vi "SMO.Dictionary.Variant.TestLauncher.vi"() -> ()   [LabVIEW 2013, in "SMO.Dictionary.lvlib" / "SMO.Dictionary.Variant.lvclass"]
uses:
  SMO.Dictionary.Variant.lvclass
  <vilib>/JKI/JKI SMO/SMO/Typedefs/SMOState --Enum.ctl
  <vilib>/JKI/JKI SMO/SMO/SMO.lvclass/SMO.ctl
  <vilib>/JKI/JKI SMO/SMO/Private/ReftoDVR--SMO.vi
  <vilib>/JKI/JKI SMO/SMO/SMO.lvclass
  SMO.Dictionary/SMO.Dictionary.lvclass
panel:
  out "deleted":bool
  in  "Delete String":bool
  out "echo":string
  out "Values":variant[](array[variant])
  in  "string":string
  in  "Update String":bool
  out "SMO State":T1
  out "error out":errorcluster
  in  "Stop":bool
  # "Variant Attributes Dictionary Test Launcher"
  # "For instructions on how to use the JKI State Machine Objects, examples and video tutorials, visit:\nhttp://jki.net/state-machine-objects/\n\nJKI State Machine Objects™\nhttp://jki.net/state-machine-objects/\nCopyright (C) 2005-2015, JKI <info@jki.net>\nALL RIGHTS RESERVED"
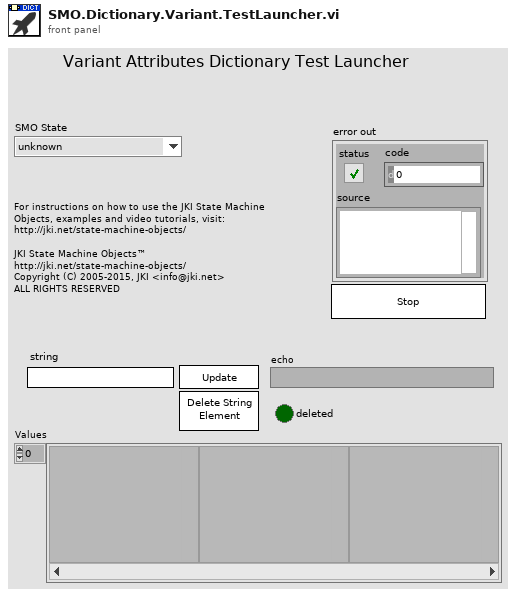
[diagram p1: front panel]
types:
  T1 = typedef "SMO.lvclass/SMOState --Enum.ctl" = enum16{"unknown", "Created", "Started", "Stopped"}
  T2 = typedef "SMO.lvclass/Public Events.ctl" = cluster{"Error":refnum<user-event>, "State":refnum<user-event>, "Reserve State":refnum<user-event>}
  T3 = typedef "SMO.Dictionary.lvlib/SMO.Dictionary.lvclass/PublicEvents--Cluster.ctl" = cluster{"Cleared":refnum<user-event>, "Deleted":refnum<user-event>, "Updated":refnum<user-event>}
  T4 = cluster{"Event Registration Refnum":refnum<event-registration>}
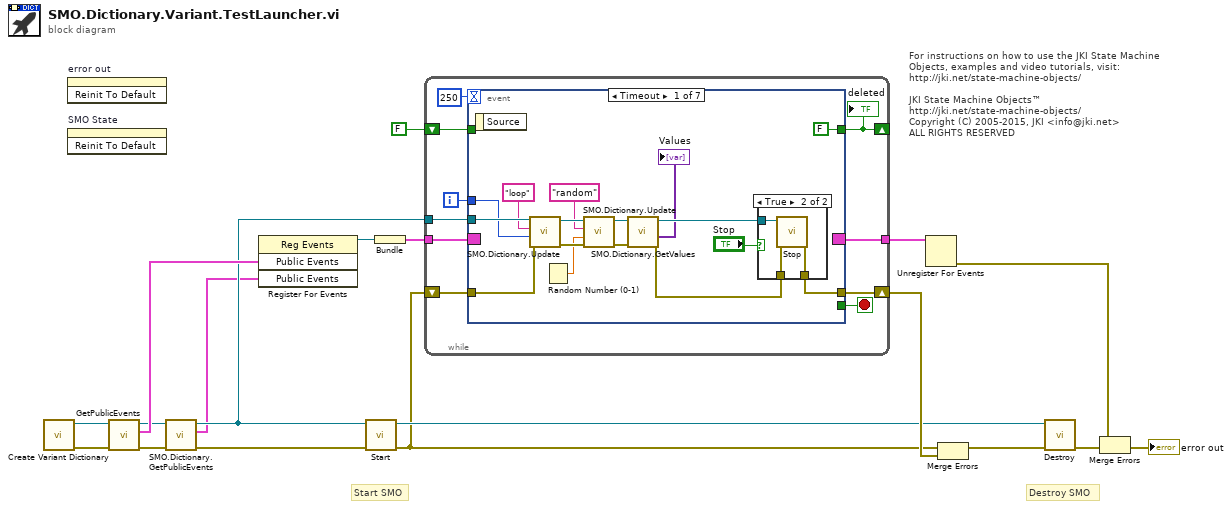
[diagram p0: block diagram]
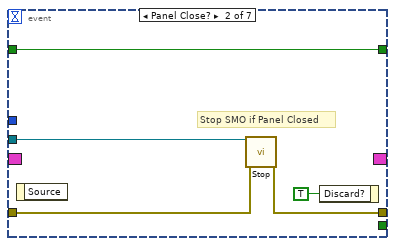
[diagram p3: hidden frame]
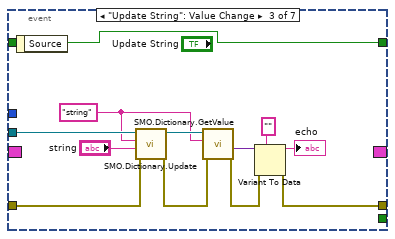
[diagram p4: hidden frame]
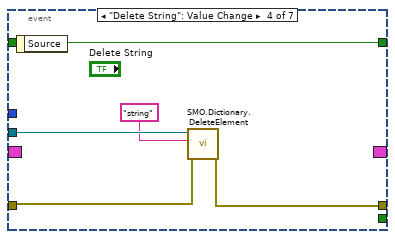
[diagram p5: hidden frame]
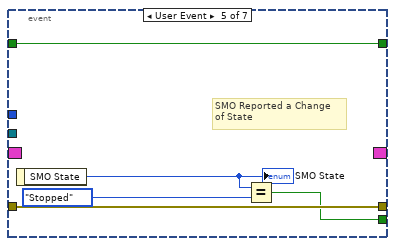
[diagram p6: hidden frame]
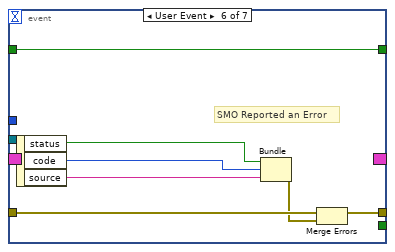
[diagram p7: hidden frame]
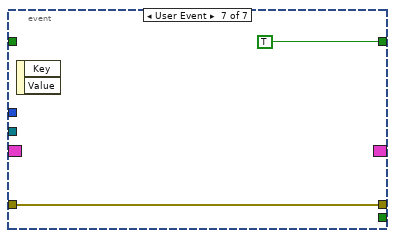
[diagram p8: hidden frame]
diagram:
  # "For instructions on how to use the JKI State Machine Objects, examples and video tutorials, visit:\nhttp://jki.net/state-machine-objects/\n\nJKI State Machine Objects™\nhttp://jki.net/state-machine-objects/\nCopyright (C) 2005-2015, JKI <info@jki.net>\nALL RIGHTS RESERVED"
  # "Start SMO"
  # "Destroy SMO"
  n1 = call "Create Variant Dictionary.vi"() -> ("error out"=w2:errorcluster, "SMO.Dictionary.Variant out"=w3:refnum<class "SMO.Dictionary.Variant.lvclass">)  [unwired: 9 in, 1 out]
  n2 = invoke on="error out" class="Clust (strict)" method="Reinit To Default"() -> ()  [unwired: 3 in, 3 out]
  n3 = invoke on="SMO State" class="Enum (strict)" method="Reinit To Default"() -> ()  [unwired: 3 in, 3 out]
  n4 = call <vilib>:"GetPublicEvents.vi"("error in (no error)"=w2, "SMO"=w3) -> ("error out"=w8:errorcluster, "Public Events"=w12:T2, "SMO out"=w10:refnum<class "SMO.Dictionary.Variant.lvclass">)  [unwired: 7 in]
  n5 = call "SMO.Dictionary.GetPublicEvents.vi"("error in (no error)"=w8, "SMO.Dictionary in"=w10) -> ("error out"=w7:errorcluster, "Public Events"=w6:T3, "SMO.Dictionary out"=w9:refnum<class "SMO.Dictionary.Variant.lvclass">)  [unwired: 7 in]
  n6 = register-events(w12, w6) -> (reference out=w11:refnum<event-registration>)  [unwired: 2 in, 1 out]
  n7 = call <vilib>:"Start.vi"("error in (no error)"=w7, "SMO"=w9) -> ("error out"=w4:errorcluster, "SMO out"=w5:refnum<class "SMO.Dictionary.Variant.lvclass">)  [unwired: 8 in]
  n8 = Bundle("Event Registration Refnum"=w11) -> (w18:T4)  [unwired: 1 in]
  n9 = while {
    shift-right: [w28] -> w17
    shift-left: w4 -> [w27]
    tunnel: w18 -> [w26]
    tunnel: [w25] -> w19
    tunnel: w9 -> [w24]
    shift-right: [w20] -> _
    shift-left: FALSE -> [w21]
    i -> [w22]
    stop <- w29 stop-if-true
    n10 = event shown="[0] Timeout" {
      selector: w26 -> [_ _ _ _ _ _ _]
      dyn-events: [_ _ _ _ _ _ _] -> w25
      timeout: 250 -> [_ _ _ _ _ _ _]
      tunnel: [_ _ _ _ w73 _ _] -> w29
      tunnel: w24 -> [w42 w54 w66 w71 _ _ _]
      tunnel: [w45 w53 w57 w68 w76 w81 w85] -> w28
      tunnel: w27 -> [w43 w52 w65 w69 w76 w79 w85]
      tunnel: w22 -> [w40 _ _ _ _ _ _]
      tunnel: w21 -> [_ w50 w55 w67 w72 w77 _]
      tunnel: [FALSE w50 w55 w67 w72 w77 TRUE] -> w20
      event Timeout {
        n11 = event-data() -> ()  [unwired: 1 in, 1 out]
        n12 = call "SMO.Dictionary.Update.vi"("error in (no error)"=w43, "Value"=w40, "Key (\"\": variant name)"="loop", "SMO.Dictionary"=w42) -> ("error out"=w39:errorcluster, "SMO.Dictionary out"=w38:refnum<class "SMO.Dictionary.Variant.lvclass">)  [unwired: 5 in, 1 out]
        n13 = Random Number (0-1)() -> (number: 0 to 1=w36:dbl)
        n14 = call "SMO.Dictionary.Update.vi"("error in (no error)"=w39, "Value"=w36, "Key (\"\": variant name)"="random", "SMO.Dictionary"=w38) -> ("error out"=w33:errorcluster, "SMO.Dictionary out"=w35:refnum<class "SMO.Dictionary.Variant.lvclass">)  [unwired: 5 in, 1 out]
        n15 = call "SMO.Dictionary.GetValues.vi"("error in (no error)"=w33, "SMO.Dictionary"=w35) -> ("error out"=w32:errorcluster, "Values"=→"Values":variant[], "SMO.Dictionary out"=w34:refnum<class "SMO.Dictionary.Variant.lvclass">)  [unwired: 5 in, 2 out]
        n16 = case shown="True" "Stop" {
          tunnel: w34 -> [_ w49]
          tunnel: [w46 w48] -> w45
          tunnel: w32 -> [w46 w47]
          frame False {
          }
          frame True {
            n17 = call <vilib>:"Stop.vi"("error in (no error)"=w47, "SMO"=w49) -> ("error out"=w48:errorcluster)  [unwired: 8 in, 1 out]
          }
        }
      }
      event Panel Close? {
        # "Stop SMO if Panel Closed"
        n18 = event-data() -> ()  [unwired: 1 in, 1 out]
        n19 = call <vilib>:"Stop.vi"("error in (no error)"=w52, "SMO"=w54) -> ("error out"=w53:errorcluster)  [unwired: 8 in, 1 out]
        n20 = event-data("Discard?"=TRUE ("OK")) -> ()  [unwired: 1 in, 1 out]
      }
      event "Update String": Value Change {
        w62 = "string"
        n21 = event-data() -> ()  [unwired: 1 in, 1 out]
        n22 = call "SMO.Dictionary.Update.vi"("error in (no error)"=w65, "Value"="string", "Key (\"\": variant name)"=w62, "SMO.Dictionary"=w66) -> ("error out"=w61:errorcluster, "SMO.Dictionary out"=w63:refnum<class "SMO.Dictionary.Variant.lvclass">)  [unwired: 5 in, 1 out]
        n23 = call "SMO.Dictionary.GetValue.vi"("error in (no error)"=w61, "Key"=w62, "SMO.Dictionary"=w63) -> ("error out"=w58:errorcluster, "Value"=w60:variant)  [unwired: 4 in, 3 out]
        n24 = Variant To Data(error in=w58, type="", Variant=w60) -> (data=→"echo":string, error out=w57:errorcluster)
      }
      event "Delete String": Value Change {
        n25 = event-data() -> ()  [unwired: 1 in, 1 out]
        n26 = call "SMO.Dictionary.DeleteElement.vi"("error in (no error)"=w69, "Key"="string", "SMO.Dictionary"=w71) -> ("error out"=w68:errorcluster)  [unwired: 6 in, 2 out]
      }
      event User Event {
        # "SMO Reported a Change\nof State"
        n27 = event-data() -> ("SMO State"=w75:T1)  [unwired: 1 in]
        "SMO State" <- w75
        n28 = Equal?(x=w75, y=SMOState_--Enum."Stopped") -> (x = y?=w73:bool)
      }
      event User Event {
        # "SMO Reported an Error"
        n29 = event-data() -> ("status"=w80:bool, "code"=w83:i32, "source"=w82:string)  [unwired: 1 in]
        n30 = Bundle("status"=w80, "code"=w83, "source"=w82) -> (w78:errorcluster)  [unwired: 1 in]
        n31 = Merge Errors(w79, w78) -> (w81:errorcluster)
      }
      event User Event {
        n32 = event-data() -> ()  [unwired: 1 in, 2 out]
      }
    }
    "deleted" <- w20
  }
  n33 = Unregister For Events(event registration refnum=w19) -> (error out=w16:errorcluster)  [unwired: 1 in]
  n34 = Merge Errors(w4, w17) -> (w13:errorcluster)
  n35 = call <vilib>:"Destroy.vi"("error in (no error)"=w13, "SMO"=w5) -> ("error out"=w14:errorcluster)  [unwired: 9 in]
  n36 = Merge Errors(w16, w14) -> (→"error out":errorcluster)
